vi "GT_CrdClear.vi"(3 "fifo in":i16, 4 "crd in":i16, 5 "rtn_In":cluster{"rtn":i16, "Func":string}) -> (0 "fifo out":i16, 1 "crd out":i16, 2 "rtn_Out":cluster{"rtn":i16, "Func":string})   [LabVIEW 2014]
uses:
  VC6/gts.dll
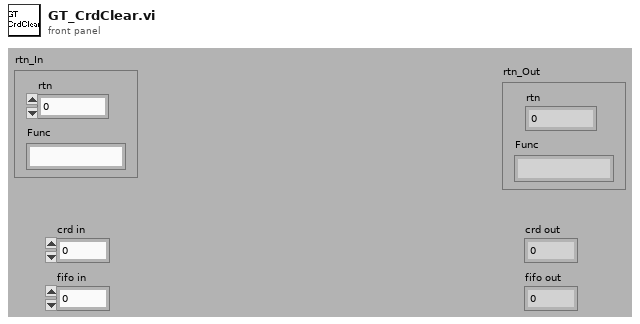
[diagram p1: front panel]
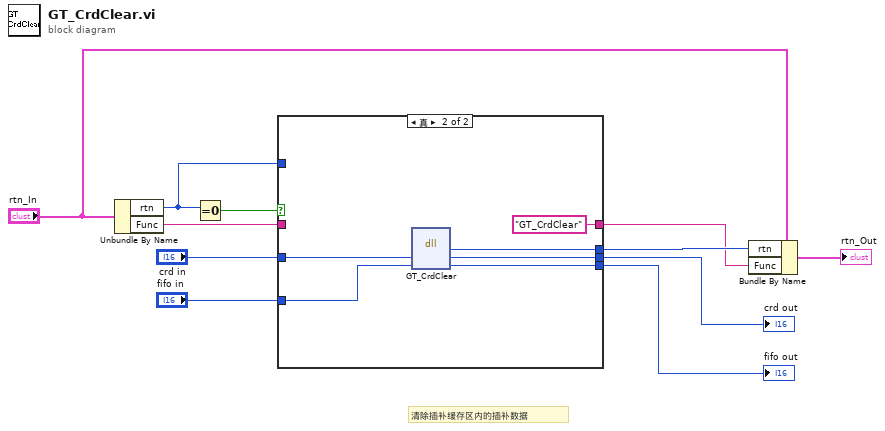
[diagram p0: block diagram]
diagram:
  # "清除插补缓存区内的插补数据"
  n1 = Unbundle By Name("rtn_In") -> ("rtn"=w3:i16, "Func"=w2:string)
  n2 = Equal To 0?(x=w3) -> (x = 0?=w11:bool)
  n3 = case shown="真" w11 {
    tunnel: "crd in" -> [w13 w21]
    tunnel: [w15 w20] -> w7
    tunnel: [w13 w19] -> w6
    tunnel: "fifo in" -> [w12 w18]
    tunnel: [w12 w17] -> w4
    tunnel: w3 -> [w15 _]
    tunnel: w2 -> [w14 _]
    tunnel: [w14 "GT_CrdClear" ("Func")] -> w1
    frame False {
    }
    frame True {
      n4 = dll-call lib="PTH2Fabs DNewGTS AC-800LWin7版源程序-20170926gts85VC6gts.dll" fn="GT_CrdClear"("crd"=w21, "fifo"=w18) -> ("rtn"=w20:i16, "crd"=w19:i16, "fifo"=w17:i16)  [unwired: 3 in, 2 out]
    }
  }
  "crd out" <- w6
  "fifo out" <- w4
  n5 = Bundle By Name(cluster="rtn_In", "rtn"=w7, "Func"=w1) -> (→"rtn_Out":cluster{"rtn":i16, "Func":string})
